vi "Destroy.vi"(8 "ErrorIn":errorcluster, 11 "YActorIn":refnum<class "YActor.lvclass">) -> (0 "ErrorOut":errorcluster, 3 "YActorOut":refnum<class "YActor.lvclass">)   [LabVIEW 2021, in "YActor.lvclass"]
uses:
  YActor.lvclass
  YActor.lvclass/YActor.ctl
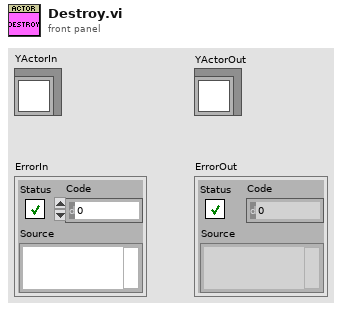
[diagram p1: front panel]
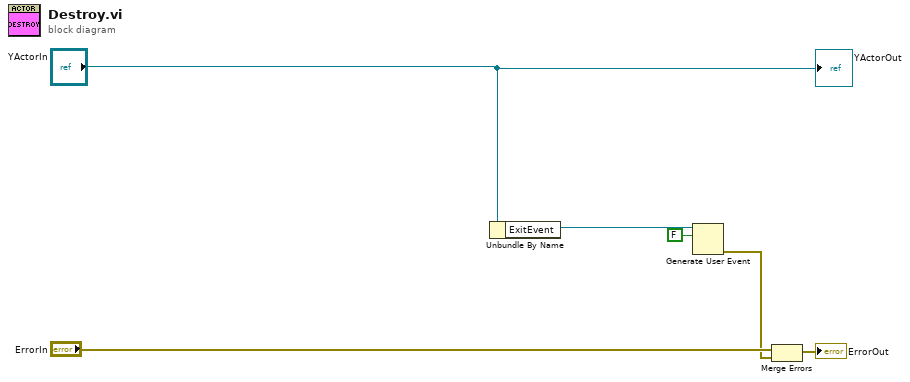
[diagram p0: block diagram]
diagram:
  n1 = Unbundle By Name("YActorIn") -> ("ExitEvent"=w3:refnum<user-event>)
  n2 = Generate User Event(user event=w3, event data cluster=FALSE ("event data")) -> (error out=w4:errorcluster)  [unwired: 2 in, 1 out]
  n3 = Merge Errors("ErrorIn", w4) -> (→"ErrorOut":errorcluster)
  "YActorOut" <- "YActorIn"
